vi "send_multipart.vi"(0 "zmq_mlt in":refnum<class "zmq_multipart_lib.lvclass">, 5 "multipart mesage in":refnum<data-value>, 9 "Enable Validaition":bool=TRUE, 11 "error in (no error)":errorcluster) -> (4 "zmq_mlt out":refnum<class "zmq_multipart_lib.lvclass">, 15 "error out":errorcluster)   [LabVIEW 2019, in "zmq_multipart_lib.lvlib" / "zmq_multipart_lib.lvclass"]
uses:
  zmq_multipart_lib.lvclass
  zmq_multipart_lib.lvclass/zmq_multipart_lib.ctl
  <vilib>/addons/zeromq/zmq_socket.lvclass
  mmw_service/src_LabVIEW/lib/mmw_Service/Service.lvlib
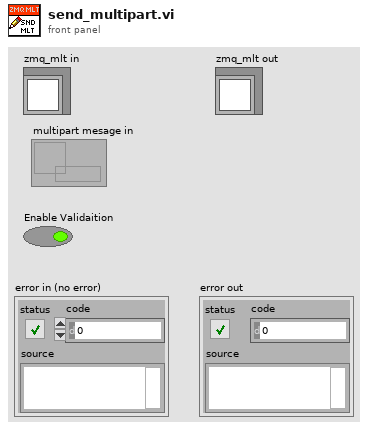
[diagram p1: front panel]
types:
  T1 = typedef "Service.lvlib/AppData.ctl" = cluster{"MsgQ":refnum<queue>, "Stop?":bool, "zmq sessions":cluster{"Control_endpoint":string, "Instr_endpoint":string}, "control-loop":cluster{"fromUI-Q":refnum<queue>, "toUI":refnum<user-event>, "Control_endpoint":string}, "UI-loop":cluster{"evnt_ref":refnum<event-registration>}, "logging":cluster{"level":dbl, "verbosity":dbl, "path":string, "Listener_ID":string}}
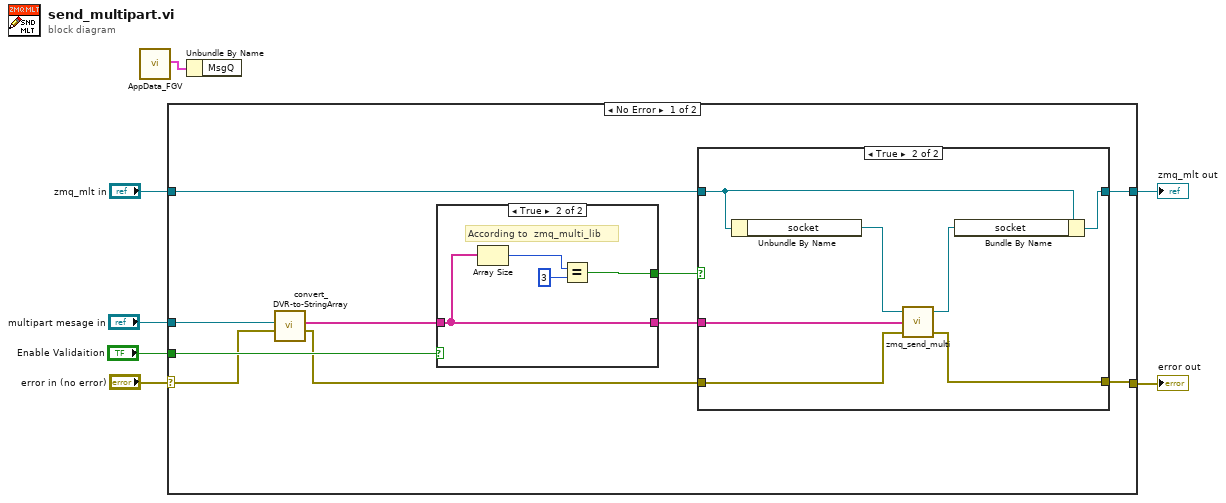
[diagram p0: block diagram]
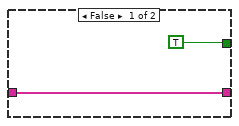
[diagram p2: hidden frame]
diagram:
  n1 = call "AppData_FGV.vi"() -> ("AppData out"=w2:T1)  [unwired: 18 in, 1 out]
  n2 = case shown="No Error" "error in (no error)" {
    selector: "error in (no error)" -> [w9 w34]
    tunnel: [w15 w34] -> w7
    tunnel: "zmq_mlt in" -> [w17 w33]
    tunnel: [w16 w33] -> w5
    tunnel: "Enable Validaition" -> [w14 _]
    tunnel: "multipart mesage in" -> [w11 _]
    frame No Error {
      n3 = call "convert_DVR-to-StringArray.vi"("error in (no error)"=w9, "multipart message DVR in"=w11) -> ("error out"=w8:errorcluster, "parts"=w10:string[])  [unwired: 6 in]
      n4 = case shown="True" w14 {
        tunnel: w10 -> [w19 w20]
        tunnel: [w19 w20] -> w13
        tunnel: [TRUE w21] -> w12
        frame False {
        }
        frame True {
          # "According to  zmq_multi_lib"
          n5 = Array Size(array=w20) -> (size(s)=w23:i32)
          n6 = Equal?(x=w23, y=3) -> (x = y?=w21:bool)
        }
      }
      n7 = case shown="True" w12 {
        tunnel: w17 -> [w25 w32]
        tunnel: [w25 w31] -> w16
        tunnel: w8 -> [w24 w28]
        tunnel: [w24 w27] -> w15
        tunnel: w13 -> [_ w26]
        frame False {
        }
        frame True {
          n8 = Unbundle By Name(w32) -> ("socket"=w30:refnum<class "zmq_socket.lvclass">)
          n9 = call <vilib>:"zmq_send_multi.vi"("error in"=w28, "parts"=w26, "socket in"=w30) -> ("error out"=w27:errorcluster, "socket out"=w29:refnum<class "zmq_socket.lvclass">)  [unwired: 1 in]
          n10 = Bundle By Name(cluster=w32, "socket"=w29) -> (w31:refnum<class "zmq_multipart_lib.lvclass">)
        }
      }
    }
    frame Error {
    }
  }
  "error out" <- w7
  "zmq_mlt out" <- w5
  n11 = Unbundle By Name(w2) -> ()  [unwired: 1 out]
